vi "UsingTheRightSenses.vi"   [LabVIEW 2014, in "LegoMindstormProjects.lvrbt"]
uses:
  LegoMindstormProjects.lvrbt
  <vilib>/NXT/Block Support/NXT_OutputPort.ctl
  <vilib>/NXT/Block Support/NXT_InputPort.ctl
  <vilib>/NXT/Subs/ColorSensorColors.ctl
  <vilib>/NXT/Dual Mode Library/Sensors/EV3_Gyro_Reset.vi
  <vilib>/NXT/NXTIO Xnodes/NXTIONodeSubVIs/NXTMoveMotors.vi
  <vilib>/NXT/Dual Mode Library/Waits/Wait_EV3_Angle_Less.vi
  <vilib>/NXT/NXTIO Xnodes/NXTIONodeSubVIs/NXTStopMotors.vi
  <vilib>/NXT/Dual Mode Library/Sensors/EV3_Color_Color.vi
  <vilib>/NXT/Dual Mode Library/Waits/Wait_EV3_Angle_Greater.vi
  <vilib>/NXT/Dual Mode Library/Waits/Wait_Rotation.vi
  <vilib>/NXT/NXTIO Xnodes/NXTIONodeSubVIs/LEGOStopAllMotors.vi
  <vilib>/NXT/Dual Mode Library/Waits/Wait_Touch.vi
  <vilib>/NXT/Dual Mode Library/Waits/Wait_Num.vi
  <vilib>/NXT/Dual Mode Library/Waits/Wait_EV3_Ultrasonic_Centimeter_Closer.vi
  <vilib>/NXT/NXTIO Xnodes/AddressXNode/NXTIOAddress.xnode
  <vilib>/NXT/NXTIO Xnodes/NXTIOXNode/NXTIO.xnode
  <vilib>/NXT/Subs/LVHSConnector.ctl
  <vilib>/NXT/LegoClasses/BrickReference/BrickReference.lvclass
types:
  T1 = typedef "NXT_InputPort.ctl" = u32
  T2 = typedef "NXT_OutputPort.ctl" = u8
  T3 = typedef "LVHSConnector.ctl" = refnum<class "BrickReference.lvclass">
  T4 = typedef "ColorSensorColors.ctl" = enum16{"No Color", "Black", "Blue", "Green", "Yellow", "Red", "White", "Brown"}
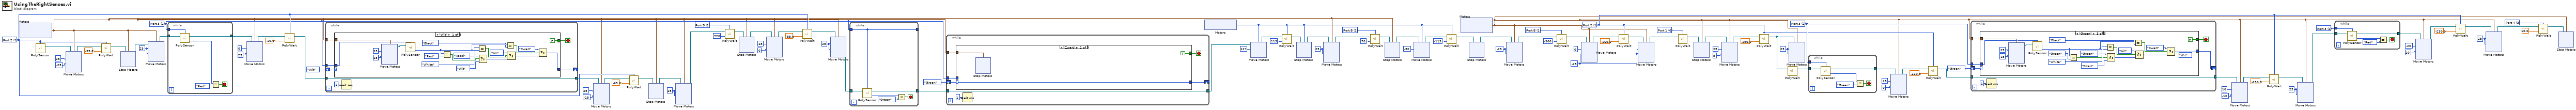
[diagram p0: block diagram]
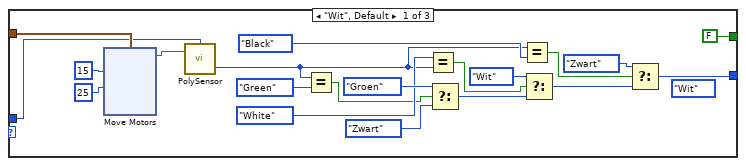
[diagram p2: hidden frame]
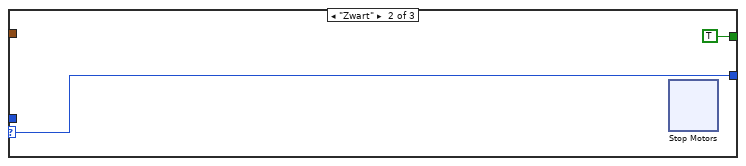
[diagram p3: hidden frame]
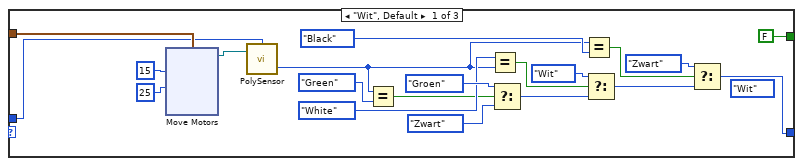
[diagram p4: hidden frame]
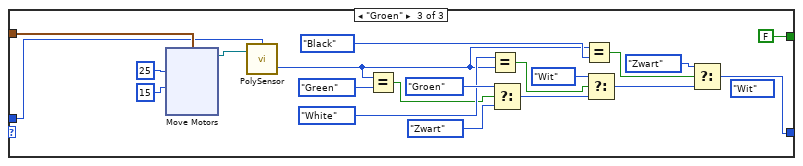
[diagram p5: hidden frame]
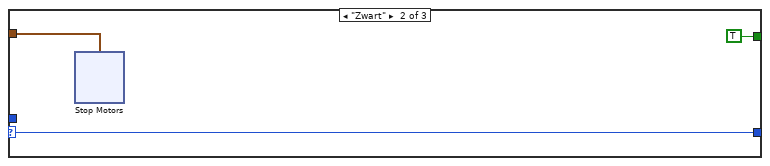
[diagram p6: hidden frame]
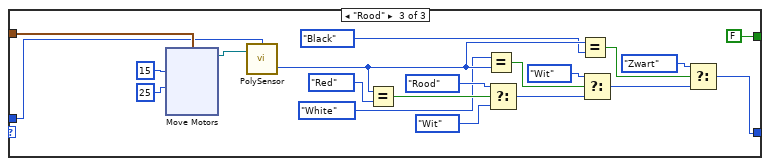
[diagram p7: hidden frame]
diagram:
  w4 = T1 3 items=["Port 1", "Port 2", "Port 3", "Port 4"] ("Port (Port 1)")
  w8 = i8 25 ("Power/Speed 1")
  w16 = T1 2 items=["Port 1", "Port 2", "Port 3", "Port 4"] ("Port (Port 1)")
  w17 = i8 25 ("Power/Speed 1")
  w30 = T1 2 items=["Port 1", "Port 2", "Port 3", "Port 4"] ("Port (Port 1)")
  w34 = i8 25 ("Power/Speed 1")
  w40 = T1 0 items=["Port 1", "Port 2", "Port 3", "Port 4"] ("Port (Port 1)")
  w9 = T1 1 items=["Port 1", "Port 2", "Port 3", "Port 4"] ("Port (Port 1)")
  w44 = i8 -25 ("Power/Speed 2")
  w50 = T2 1 items=["Port A", "Port B", "Port C", "Port D"] ("Port (Port A)")
  w52 = i8 -25 ("Power/Speed 2")
  w63 = T2 1 items=["Port A", "Port B", "Port C", "Port D"] ("Port (Port A)")
  w64 = i8 25 ("Power/Speed 2")
  w78 = i8 25 ("Power/Speed 1")
  w89 = T2 1 items=["Port A", "Port B", "Port C", "Port D"] ("Port (Port A)")
  w90 = i8 25 ("Power/Speed 1")
  w104 = i8 25 ("Power/Speed 1")
  w79 = T1 1 items=["Port 1", "Port 2", "Port 3", "Port 4"] ("Port (Port 1)")
  w73 = T1 2 items=["Port 1", "Port 2", "Port 3", "Port 4"] ("Port (Port 1)")
  n1 = xnode "Motors"() -> ("Motor"=w60:cluster{"Port":T2, "Port":T2})
  n2 = call-poly <vilib>:"PolySensor.vi"("Port (Port 1)"=w79) -> ("NXT/EV3"=w109:T3)  [unwired: 3 in]
  n3 = xnode "Move Motors"("Power/Speed 2"=i8 -25, "Power/Speed 1"=i8 25, "Motors"=w60, "NXT/EV3"=w109) -> ("NXT/EV3"=w106:T3)
  n4 = call-poly <vilib>:"PolyWait.vi"("Degrees (180)"=sgl -35.0, "NXT/EV3"=w106, "Port (Port 1)"=w79) -> ("NXT/EV3"=w103:T3)  [unwired: 1 in]
  n5 = xnode "Stop Motors"("Motors"=w60, "NXT/EV3"=w103) -> ("NXT/EV3"=w102:T3)
  n6 = xnode "Move Motors"("Power/Speed 2"=w104, "Power/Speed 1"=w104, "Motors"=w60, "NXT/EV3"=w102) -> ("NXT/EV3"=w76:T3)
  n7 = while {
    tunnel: w73 -> [w116]
    tunnel: w76 -> [w112]
    tunnel: [w111] -> w75
    stop <- w113 stop-if-true
    n8 = call-poly <vilib>:"PolySensor.vi"("NXT/EV3"=w112, "Port (Port 1)"=w116) -> ("Detected Color"=w115:T4, "NXT/EV3"=w111:T3)  [unwired: 1 in]
    n9 = Equal?(x=w115, y=ColorSensorColors."Red") -> (x = y?=w113:bool)
  }
  n10 = xnode "Move Motors"("Power/Speed 2"=i8 25, "Power/Speed 1"=i8 0, "Motors"=w60, "NXT/EV3"=w75) -> ("NXT/EV3"=w99:T3)
  n11 = call-poly <vilib>:"PolyWait.vi"("Degrees (180)"=sgl -10.0, "NXT/EV3"=w99, "Port (Port 1)"=w79) -> ("NXT/EV3"=w98:T3)  [unwired: 1 in]
  n12 = while {
    shift-right: [w120] -> _
    shift-left: enum16{"Wit", "Zwart", "Rood"}."Wit" ("Enum") -> [w123]
    tunnel: w60 -> [w122]
    tunnel: w73 -> [w119]
    tunnel: w98 -> [w117]
    tunnel: [w117] -> w77
    stop <- w118 stop-if-true
    n13 = case shown="\"Wit\"" w123 {
      selector: w123 -> [_ w153 _]
      tunnel: w122 -> [w128 w152 w179]
      tunnel: w119 -> [w127 _ w175]
      tunnel: [w124 w153 w163] -> w120
      tunnel: [FALSE TRUE FALSE] -> w118
      frame "Wit" {
        n14 = xnode "Move Motors"("Power/Speed 2"=i8 15, "Power/Speed 1"=i8 25 ("Power/Speed 2"), "Motors"=w128) -> ("NXT/EV3"=w142:T3)  [unwired: 1 in]
        n15 = call-poly <vilib>:"PolySensor.vi"("NXT/EV3"=w142, "Port (Port 1)"=w127) -> ("Detected Color"=w136:T4)  [unwired: 1 in, 1 out]
        n16 = Equal?(x=w136, y=ColorSensorColors."Red") -> (x = y?=w140:bool)
        n17 = Equal?(x=ColorSensorColors."White" ("y"), y=w136) -> (x = y?=w137:bool)
        n18 = Select(t=enum16{"Wit", "Zwart", "Rood"}."Rood" ("Enum"), s=w140, f=enum16{"Wit", "Zwart", "Rood"}."Wit" ("Enum")) -> (s? t:f=w138:enum16{"Wit", "Zwart", "Rood"})
        n19 = Equal?(x=w136, y=ColorSensorColors."Black") -> (x = y?=w135:bool)
        n20 = Select(t=enum16{"Wit", "Zwart", "Rood"}."Wit" ("Enum"), s=w137, f=w138) -> (s? t:f=w134:enum16{"Wit", "Zwart", "Rood"})
        n21 = Select(t=enum16{"Wit", "Zwart", "Rood"}."Zwart" ("Enum"), s=w135, f=w134) -> (s? t:f=w124:enum16{"Wit", "Zwart", "Rood"})
      }
      frame "Zwart" {
        n22 = xnode "Stop Motors"("Motors"=w152) -> ()  [unwired: 1 in, 1 out]
      }
      frame "Rood" {
        n23 = xnode "Move Motors"("Power/Speed 2"=i8 25, "Power/Speed 1"=i8 15 ("Power/Speed 2"), "Motors"=w179) -> ("NXT/EV3"=w176:T3)  [unwired: 1 in]
        n24 = call-poly <vilib>:"PolySensor.vi"("NXT/EV3"=w176, "Port (Port 1)"=w175) -> ("Detected Color"=w169:T4)  [unwired: 1 in, 1 out]
        n25 = Equal?(x=w169, y=ColorSensorColors."Red") -> (x = y?=w173:bool)
        n26 = Equal?(x=ColorSensorColors."White" ("y"), y=w169) -> (x = y?=w170:bool)
        n27 = Select(t=enum16{"Wit", "Zwart", "Rood"}."Rood" ("Enum"), s=w173, f=enum16{"Wit", "Zwart", "Rood"}."Wit" ("Enum")) -> (s? t:f=w171:enum16{"Wit", "Zwart", "Rood"})
        n28 = Equal?(x=w169, y=ColorSensorColors."Black") -> (x = y?=w168:bool)
        n29 = Select(t=enum16{"Wit", "Zwart", "Rood"}."Wit" ("Enum"), s=w170, f=w171) -> (s? t:f=w167:enum16{"Wit", "Zwart", "Rood"})
        n30 = Select(t=enum16{"Wit", "Zwart", "Rood"}."Zwart" ("Enum"), s=w168, f=w167) -> (s? t:f=w163:enum16{"Wit", "Zwart", "Rood"})
      }
    }
    n31 = Wait (ms)(milliseconds to wait=u32 1) -> ()  [unwired: 1 out]
  }
  n32 = xnode "Move Motors"("Power/Speed 2"=i8 -25, "Power/Speed 1"=i8 25, "Motors"=w60, "NXT/EV3"=w77) -> ("NXT/EV3"=w93:T3)
  n33 = call-poly <vilib>:"PolyWait.vi"("Degrees (180)"=sgl -65.0, "NXT/EV3"=w93, "Port (Port 1)"=w79) -> ("NXT/EV3"=w92:T3)  [unwired: 1 in]
  n34 = xnode "Stop Motors"("Motors"=w60, "NXT/EV3"=w92) -> ("NXT/EV3"=w91:T3)
  n35 = xnode "Move Motors"("Power/Speed 2"=w90, "Power/Speed 1"=w90, "Motors"=w60, "NXT/EV3"=w91) -> ("NXT/EV3"=w88:T3)
  n36 = call-poly <vilib>:"PolyWait.vi"("Position Change (180)"=720, "NXT/EV3"=w88, "Port (Port A)"=w89) -> ("NXT/EV3"=w86:T3)  [unwired: 1 in]
  n37 = xnode "Stop Motors"("Motors"=w60, "NXT/EV3"=w86) -> ("NXT/EV3"=w85:T3)
  n38 = xnode "Move Motors"("Power/Speed 2"=i8 0, "Power/Speed 1"=i8 25, "Motors"=w60, "NXT/EV3"=w85) -> ("NXT/EV3"=w81:T3)
  n39 = call-poly <vilib>:"PolyWait.vi"("Degrees (180)"=sgl -85.0, "NXT/EV3"=w81, "Port (Port 1)"=w79) -> ("NXT/EV3"=w80:T3)  [unwired: 1 in]
  n40 = xnode "Move Motors"("Power/Speed 2"=w78, "Power/Speed 1"=w78, "Motors"=w60, "NXT/EV3"=w80) -> ("NXT/EV3"=w74:T3)
  n41 = while {
    tunnel: [w188] -> _
    tunnel: w74 -> [w190]
    tunnel: [w189] -> w71
    tunnel: w73 -> [w188]
    stop <- w191 stop-if-true
    n42 = call-poly <vilib>:"PolySensor.vi"("NXT/EV3"=w190, "Port (Port 1)"=w188) -> ("Detected Color"=w193:T4, "NXT/EV3"=w189:T3)  [unwired: 1 in]
    n43 = Equal?(x=w193, y=ColorSensorColors."Green") -> (x = y?=w191:bool)
  }
  n44 = while {
    tunnel: w60 -> [w199]
    tunnel: w73 -> [w198]
    shift-right: [w196] -> _
    shift-left: enum16{"Wit", "Zwart", "Groen"}."Groen" ("Enum") -> [w197]
    tunnel: w71 -> [w194]
    tunnel: [w194] -> w70
    stop <- w195 stop-if-true
    n45 = case shown="\"Zwart\"" w197 {
      selector: w197 -> [_ w229 _]
      tunnel: w199 -> [w205 w231 w241]
      tunnel: w198 -> [w201 _ w240]
      tunnel: [w203 w229 w238] -> w196
      tunnel: [FALSE TRUE FALSE] -> w195
      frame "Wit", Default {
        (unwired) enum16{"Wit", "Zwart", "Groen"}."Wit" ("Enum")
        n46 = xnode "Move Motors"("Power/Speed 2"=i8 25, "Power/Speed 1"=i8 15 ("Power/Speed 2"), "Motors"=w205) -> ("NXT/EV3"=w207:T3)  [unwired: 1 in]
        n47 = call-poly <vilib>:"PolySensor.vi"("NXT/EV3"=w207, "Port (Port 1)"=w201) -> ("Detected Color"=w212:T4)  [unwired: 1 in, 1 out]
        n48 = Equal?(x=w212, y=ColorSensorColors."Green") -> (x = y?=w209:bool)
        n49 = Equal?(x=ColorSensorColors."White" ("y"), y=w212) -> (x = y?=w211:bool)
        n50 = Select(t=enum16{"Wit", "Zwart", "Groen"}."Groen" ("Enum"), s=w209, f=enum16{"Wit", "Zwart", "Groen"}."Zwart" ("Enum")) -> (s? t:f=w210:enum16{"Wit", "Zwart", "Groen"})
        n51 = Equal?(x=w212, y=ColorSensorColors."Black") -> (x = y?=w213:bool)
        n52 = Select(t=enum16{"Wit", "Zwart", "Groen"}."Wit" ("Enum"), s=w211, f=w210) -> (s? t:f=w214:enum16{"Wit", "Zwart", "Groen"})
        n53 = Select(t=enum16{"Wit", "Zwart", "Groen"}."Zwart" ("Enum"), s=w213, f=w214) -> (s? t:f=w203:enum16{"Wit", "Zwart", "Groen"})
      }
      frame "Zwart" {
        n54 = xnode "Stop Motors"("Motors"=w231) -> ()  [unwired: 1 in, 1 out]
      }
      frame "Groen" {
        (unwired) enum16{"Wit", "Zwart", "Groen"}."Wit" ("Enum")
        n55 = xnode "Move Motors"("Power/Speed 2"=i8 15, "Power/Speed 1"=i8 25 ("Power/Speed 2"), "Motors"=w241) -> ("NXT/EV3"=w243:T3)  [unwired: 1 in]
        n56 = call-poly <vilib>:"PolySensor.vi"("NXT/EV3"=w243, "Port (Port 1)"=w240) -> ("Detected Color"=w248:T4)  [unwired: 1 in, 1 out]
        n57 = Equal?(x=w248, y=ColorSensorColors."Green") -> (x = y?=w245:bool)
        n58 = Equal?(x=ColorSensorColors."White" ("y"), y=w248) -> (x = y?=w247:bool)
        n59 = Select(t=enum16{"Wit", "Zwart", "Groen"}."Groen" ("Enum"), s=w245, f=enum16{"Wit", "Zwart", "Groen"}."Zwart" ("Enum")) -> (s? t:f=w246:enum16{"Wit", "Zwart", "Groen"})
        n60 = Equal?(x=w248, y=ColorSensorColors."Black") -> (x = y?=w249:bool)
        n61 = Select(t=enum16{"Wit", "Zwart", "Groen"}."Wit" ("Enum"), s=w247, f=w246) -> (s? t:f=w250:enum16{"Wit", "Zwart", "Groen"})
        n62 = Select(t=enum16{"Wit", "Zwart", "Groen"}."Zwart" ("Enum"), s=w249, f=w250) -> (s? t:f=w238:enum16{"Wit", "Zwart", "Groen"})
      }
    }
    n63 = Wait (ms)(milliseconds to wait=u32 1) -> ()  [unwired: 1 out]
  }
  n64 = xnode "Motors"() -> ("Motor"=w54:T2)
  n65 = xnode "Move Motors"("Power/Speed 1"=i8 127, "Motors"=w54, "NXT/EV3"=w70) -> ("NXT/EV3"=w68:T3)
  n66 = call-poly <vilib>:"PolyWait.vi"("Position Change (180)"=115, "NXT/EV3"=w68, "Port (Port A)"=w54) -> ("NXT/EV3"=w66:T3)  [unwired: 1 in]
  n67 = xnode "Stop Motors"("Motors"=w54, "NXT/EV3"=w66) -> ("NXT/EV3"=w65:T3)
  n68 = xnode "Move Motors"("Power/Speed 2"=w64, "Power/Speed 1"=w64, "Motors"=w60, "NXT/EV3"=w65) -> ("NXT/EV3"=w62:T3)
  n69 = call-poly <vilib>:"PolyWait.vi"("Position Change (180)"=70, "NXT/EV3"=w62, "Port (Port A)"=w63) -> ("NXT/EV3"=w59:T3)  [unwired: 1 in]
  n70 = xnode "Stop Motors"("Motors"=w60, "NXT/EV3"=w59) -> ("NXT/EV3"=w58:T3)
  n71 = xnode "Move Motors"("Power/Speed 1"=i8 -50, "Motors"=w54, "NXT/EV3"=w58) -> ("NXT/EV3"=w56:T3)
  n72 = call-poly <vilib>:"PolyWait.vi"("Position Change (180)"=-115, "NXT/EV3"=w56, "Port (Port A)"=w54) -> ("NXT/EV3"=w53:T3)  [unwired: 1 in]
  n73 = xnode "Motors"() -> ("Motor"=w2:cluster{"Port":T2, "Port":T2})
  n74 = xnode "Stop Motors"("NXT/EV3"=w53) -> ("NXT/EV3"=w1:T3)  [unwired: 1 in]
  n75 = xnode "Move Motors"("Power/Speed 2"=w52, "Power/Speed 1"=w52, "Motors"=w2, "NXT/EV3"=w1) -> ("NXT/EV3"=w51:T3)
  n76 = call-poly <vilib>:"PolyWait.vi"("Position Change (180)"=-900, "NXT/EV3"=w51, "Port (Port A)"=w50) -> ("NXT/EV3"=w48:T3)  [unwired: 1 in]
  n77 = xnode "Move Motors"("Power/Speed 2"=w44, "Power/Speed 1"=i8 0, "Motors"=w2, "NXT/EV3"=w48) -> ("NXT/EV3"=w46:T3)
  n78 = call-poly <vilib>:"PolyWait.vi"("Degrees (180)"=sgl -160.0, "NXT/EV3"=w46, "Port (Port 1)"=w9) -> ("NXT/EV3"=w43:T3)  [unwired: 1 in]
  n79 = xnode "Move Motors"("Power/Speed 2"=w44, "Power/Speed 1"=w44, "Motors"=w2, "NXT/EV3"=w43) -> ("NXT/EV3"=w42:T3)
  n80 = call-poly <vilib>:"PolyWait.vi"("NXT/EV3"=w42, "Port (Port 1)"=w40) -> ("NXT/EV3"=w41:T3)  [unwired: 2 in]
  n81 = xnode "Stop Motors"("Motors"=w2, "NXT/EV3"=w41) -> ("NXT/EV3"=w39:T3)
  n82 = xnode "Move Motors"("Power/Speed 2"=i8 5, "Power/Speed 1"=i8 25, "Motors"=w2, "NXT/EV3"=w39) -> ("NXT/EV3"=w36:T3)
  n83 = call-poly <vilib>:"PolyWait.vi"("Degrees (180)"=sgl -190.0, "NXT/EV3"=w36, "Port (Port 1)"=w9) -> ("NXT/EV3"=w33:T3)  [unwired: 1 in]
  n84 = call-poly <vilib>:"PolyWait.vi"("NXT/EV3"=w33) -> ("NXT/EV3"=w32:T3)  [unwired: 3 in]
  n85 = xnode "Move Motors"("Power/Speed 2"=w34, "Power/Speed 1"=w34, "Motors"=w2, "NXT/EV3"=w33) -> ()  [unwired: 1 out]
  n86 = while {
    tunnel: w32 -> [w268]
    tunnel: w30 -> [w267]
    tunnel: [w265] -> w29
    stop <- w266 stop-if-true
    n87 = call-poly <vilib>:"PolySensor.vi"("NXT/EV3"=w268, "Port (Port 1)"=w267) -> ("Detected Color"=w270:T4, "NXT/EV3"=w265:T3)  [unwired: 1 in]
    n88 = Equal?(x=w270, y=ColorSensorColors."Green") -> (x = y?=w266:bool)
  }
  n89 = xnode "Move Motors"("Power/Speed 2"=i8 0, "Power/Speed 1"=i8 25, "Motors"=w2, "NXT/EV3"=w29) -> ("NXT/EV3"=w26:T3)
  n90 = call-poly <vilib>:"PolyWait.vi"("Degrees (180)"=sgl -220.0, "NXT/EV3"=w26, "Port (Port 1)"=w9) -> ("NXT/EV3"=w24:T3)  [unwired: 1 in]
  n91 = while {
    shift-right: [w275] -> _
    shift-left: enum16{"Wit", "Zwart", "Groen"}."Groen" ("Enum") -> [w276]
    tunnel: w2 -> [w273]
    tunnel: w30 -> [w272]
    tunnel: w24 -> [w271]
    tunnel: [w271] -> w23
    stop <- w274 stop-if-true
    n92 = case shown="\"Groen\"" w276 {
      selector: w276 -> [_ w306 _]
      tunnel: [w282 w306 w317] -> w275
      tunnel: [FALSE TRUE FALSE] -> w274
      tunnel: w273 -> [w280 _ w315]
      tunnel: w272 -> [w278 _ w313]
      frame "Wit", Default {
        (unwired) enum16{"Wit", "Zwart", "Groen"}."Wit" ("Enum")
        n93 = xnode "Move Motors"("Power/Speed 2"=i8 25, "Power/Speed 1"=i8 15 ("Power/Speed 2"), "Motors"=w280) -> ("NXT/EV3"=w284:T3)  [unwired: 1 in]
        n94 = call-poly <vilib>:"PolySensor.vi"("NXT/EV3"=w284, "Port (Port 1)"=w278) -> ("Detected Color"=w289:T4)  [unwired: 1 in, 1 out]
        n95 = Equal?(x=w289, y=ColorSensorColors."Green") -> (x = y?=w286:bool)
        n96 = Equal?(x=ColorSensorColors."White" ("y"), y=w289) -> (x = y?=w288:bool)
        n97 = Select(t=enum16{"Wit", "Zwart", "Groen"}."Groen" ("Enum"), s=w286, f=enum16{"Wit", "Zwart", "Groen"}."Zwart" ("Enum")) -> (s? t:f=w287:enum16{"Wit", "Zwart", "Groen"})
        n98 = Equal?(x=w289, y=ColorSensorColors."Black") -> (x = y?=w290:bool)
        n99 = Select(t=enum16{"Wit", "Zwart", "Groen"}."Wit" ("Enum"), s=w288, f=w287) -> (s? t:f=w291:enum16{"Wit", "Zwart", "Groen"})
        n100 = Select(t=enum16{"Wit", "Zwart", "Groen"}."Zwart" ("Enum"), s=w290, f=w291) -> (s? t:f=w282:enum16{"Wit", "Zwart", "Groen"})
      }
      frame "Zwart" {
        n101 = xnode "Stop Motors"() -> ()  [unwired: 2 in, 1 out]
      }
      frame "Groen" {
        (unwired) enum16{"Wit", "Zwart", "Groen"}."Wit" ("Enum")
        n102 = xnode "Move Motors"("Power/Speed 2"=i8 15, "Power/Speed 1"=i8 25 ("Power/Speed 2"), "Motors"=w315) -> ("NXT/EV3"=w319:T3)  [unwired: 1 in]
        n103 = call-poly <vilib>:"PolySensor.vi"("NXT/EV3"=w319, "Port (Port 1)"=w313) -> ("Detected Color"=w324:T4)  [unwired: 1 in, 1 out]
        n104 = Equal?(x=w324, y=ColorSensorColors."Green") -> (x = y?=w321:bool)
        n105 = Equal?(x=ColorSensorColors."White" ("y"), y=w324) -> (x = y?=w323:bool)
        n106 = Select(t=enum16{"Wit", "Zwart", "Groen"}."Groen" ("Enum"), s=w321, f=enum16{"Wit", "Zwart", "Groen"}."Zwart" ("Enum")) -> (s? t:f=w322:enum16{"Wit", "Zwart", "Groen"})
        n107 = Equal?(x=w324, y=ColorSensorColors."Black") -> (x = y?=w325:bool)
        n108 = Select(t=enum16{"Wit", "Zwart", "Groen"}."Wit" ("Enum"), s=w323, f=w322) -> (s? t:f=w326:enum16{"Wit", "Zwart", "Groen"})
        n109 = Select(t=enum16{"Wit", "Zwart", "Groen"}."Zwart" ("Enum"), s=w325, f=w326) -> (s? t:f=w317:enum16{"Wit", "Zwart", "Groen"})
      }
    }
    n110 = Wait (ms)(milliseconds to wait=u32 1) -> ()  [unwired: 1 out]
  }
  n111 = xnode "Move Motors"("Power/Speed 2"=i8 -10, "Power/Speed 1"=i8 10, "Motors"=w2, "NXT/EV3"=w23) -> ("NXT/EV3"=w20:T3)
  n112 = call-poly <vilib>:"PolyWait.vi"("Degrees (180)"=sgl -250.0, "NXT/EV3"=w20, "Port (Port 1)"=w9) -> ("NXT/EV3"=w18:T3)  [unwired: 1 in]
  n113 = xnode "Move Motors"("Power/Speed 2"=w17, "Power/Speed 1"=w17, "Motors"=w2, "NXT/EV3"=w18) -> ("NXT/EV3"=w15:T3)
  n114 = while {
    tunnel: w15 -> [w344]
    tunnel: w16 -> [w343]
    tunnel: [w341] -> w14
    stop <- w342 stop-if-true
    n115 = call-poly <vilib>:"PolySensor.vi"("NXT/EV3"=w344, "Port (Port 1)"=w343) -> ("Detected Color"=w346:T4, "NXT/EV3"=w341:T3)  [unwired: 1 in]
    n116 = Equal?(x=w346, y=ColorSensorColors."Red") -> (x = y?=w342:bool)
  }
  n117 = xnode "Move Motors"("Power/Speed 2"=i8 20, "Power/Speed 1"=i8 -20, "Motors"=w2, "NXT/EV3"=w14) -> ("NXT/EV3"=w11:T3)
  n118 = call-poly <vilib>:"PolyWait.vi"("Degrees (180)"=sgl -230.0, "NXT/EV3"=w11, "Port (Port 1)"=w9) -> ("NXT/EV3"=w7:T3)  [unwired: 1 in]
  n119 = xnode "Move Motors"("Power/Speed 2"=w8, "Power/Speed 1"=w8, "Motors"=w2, "NXT/EV3"=w7) -> ("NXT/EV3"=w5:T3)
  n120 = call-poly <vilib>:"PolyWait.vi"("Centimeters (40)"=sgl 10.0, "NXT/EV3"=w5, "Port (Port 1)"=w4) -> ("NXT/EV3"=w3:T3)  [unwired: 1 in]
  n121 = xnode "Stop Motors"("Motors"=w2, "NXT/EV3"=w3) -> ()  [unwired: 1 out]
